vi "콜라 자판기(생산자소비자).vi"() -> ()   [LabVIEW 2018]
panel:
  out "Count Up":i32
  in  "종료":bool
  in  "반환":bool
  in  "구매":bool
  in  "동전":cluster{bool, bool, bool, bool}
  out "투입 금액":dbl
  out "링":u16(ring)
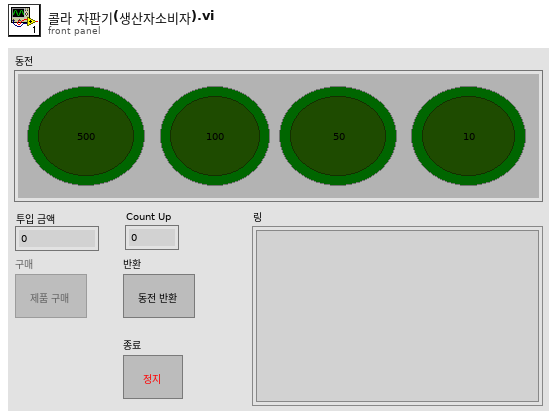
[diagram p1: front panel]
types:
  T1 = enum8{"Enabled", "Disabled", "Disabled and Grayed Out"}
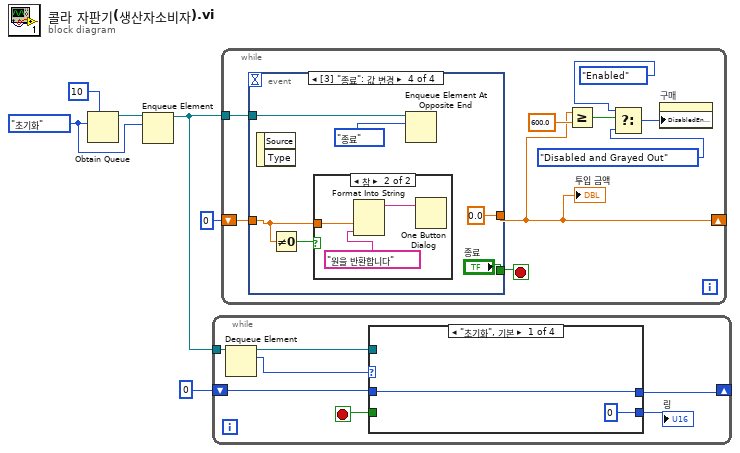
[diagram p0: block diagram]
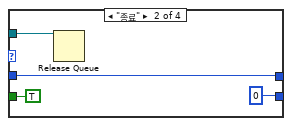
[diagram p2: hidden frame]
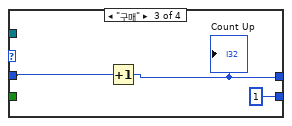
[diagram p3: hidden frame]
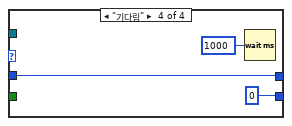
[diagram p4: hidden frame]
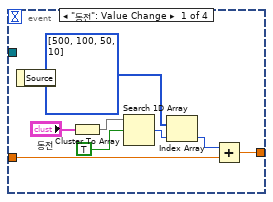
[diagram p5: hidden frame]
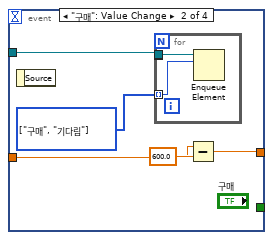
[diagram p6: hidden frame]
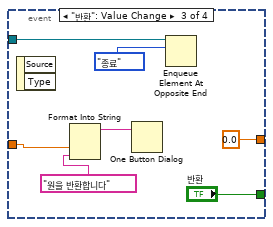
[diagram p7: hidden frame]
diagram:
  w4 = enum16{"Idle", "초기화", "종료", "구매", "반환", "기다림"}."초기화" ("열거형")
  n1 = Obtain Queue(max queue size (-1, unlimited)=10 ("최대 큐 크기(-1,제한없음)"), element data type=w4) -> (queue out=w3:refnum<queue>)  [unwired: 3 in, 2 out]
  n2 = Enqueue Element(queue=w3, element=w4) -> (queue out=w2:refnum<queue>)  [unwired: 2 in, 2 out]
  n3 = while {
    shift-right: [w8] -> _
    shift-left: 0 -> [w9]
    tunnel: w2 -> [w13]
    stop <- w7 stop-if-true
    n4 = Dequeue Element(queue=w13) -> (queue out=w11:refnum<queue>, element=w12:enum16{"Idle", "초기화", "종료", "구매", "반환", "기다림"})  [unwired: 2 in, 2 out]
    n5 = case shown="\"초기화\", 기본" w12 {
      tunnel: w11 -> [_ w18 _ _]
      tunnel: [0 0 1 0] -> w10
      tunnel: w9 -> [w14 w16 w22 w25]
      tunnel: [w14 w16 w20 w25] -> w8
      tunnel: [_ TRUE _ _] -> w7
      frame "초기화", Default {
      }
      frame "종료" {
        n6 = Release Queue(queue=w18) -> ()  [unwired: 2 in, 3 out]
      }
      frame "구매" {
        n7 = Increment(x=w22) -> (x+1=w20:i32)
        "Count Up" <- w20
      }
      frame "기다림" {
        n8 = Wait (ms)(milliseconds to wait=u32 1000 ("대기 시간 (ms)")) -> ()  [unwired: 1 out]
      }
    }
    "링" <- w10
  }
  n9 = while {
    shift-right: [w32] -> _
    shift-left: 0 -> [w34]
    tunnel: w2 -> [w27]
    stop <- w26 stop-if-true
    n10 = event shown="[3] \"종료\": 값 변경" {
      selector: _ -> [_ _ _ _]
      dyn-events: _ -> [_ _ _ _]
      timeout: _ -> [_ _ _ _]
      tunnel: [w36 w45 0.0 0.0] -> w32
      tunnel: w34 -> [w35 w46 w52 w57]
      tunnel: w27 -> [_ w44 w55 w62]
      tunnel: [_ _ "반환" "종료"] -> w26
      event "동전": Value Change {
        n11 = event-data() -> ()  [unwired: 1 in, 1 out]
        n12 = Cluster To Array(cluster="동전") -> (array=w41:bool[])
        n13 = Search 1D Array(1D array=w41, element=TRUE ("원소")) -> (index of element=w39:i32)  [unwired: 1 in]
        n14 = Index Array(array=i32[] [500, 100, 50, 10], index=w39) -> (element=w37:i32)
        n15 = Add(x=w37, y=w35) -> (x+y=w36:dbl)
      }
      event "구매": Value Change {
        w43 = enum16{"Idle", "초기화", "종료", "구매", "반환", "기다림"}[] [enum."구매", enum."기다림"] items=["Idle", "초기화", "종료", "구매", "반환", "기다림"]
        n16 = event-data() -> ()  [unwired: 1 in, 1 out]
        n17 = for {
          tunnel: [w49] -> _ mode=indexing
          tunnel: w44 -> [w49]
          tunnel: w43 -> [w48] mode=indexing
          n18 = Enqueue Element(queue=w49, element=w48) -> ()  [unwired: 2 in, 3 out]
        }
        n19 = Subtract(x=w46, y=600.0) -> (x-y=w45:dbl)
      }
      event "반환": Value Change {
        n20 = event-data() -> ()  [unwired: 1 in, 2 out]
        n21 = Format Into String(w52, "원을 반환합니다") -> (resulting string=w50:string)  [unwired: 3 in, 1 out]
        n22 = One Button Dialog(message=w50) -> ()  [unwired: 1 in, 1 out]
        n23 = Enqueue Element At Opposite End(queue=w55, element=enum16{"Idle", "초기화", "종료", "구매", "반환", "기다림"}."종료" ("열거형")) -> ()  [unwired: 2 in, 3 out]
      }
      event "종료": Value Change {
        n24 = event-data() -> ()  [unwired: 1 in, 2 out]
        n25 = Not Equal To 0?(x=w57) -> (x != 0?=w58:bool)
        n26 = case shown="참" w58 {
          tunnel: w57 -> [_ w65]
          frame False {
          }
          frame True {
            n27 = Format Into String(w65, "원을 반환합니다") -> (resulting string=w63:string)  [unwired: 3 in, 1 out]
            n28 = One Button Dialog(message=w63) -> ()  [unwired: 1 in, 1 out]
          }
        }
        n29 = Enqueue Element At Opposite End(queue=w62, element=enum16{"Idle", "초기화", "종료", "구매", "반환", "기다림"}."종료" ("열거형")) -> ()  [unwired: 2 in, 3 out]
      }
    }
    "투입 금액" <- w32
    n30 = Greater Or Equal?(x=w32, y=600.0) -> (x >= y?=w31:bool)
    n31 = Select(t=T1."Enabled" ("비활성화"), s=w31, f=T1."Disabled and Grayed Out" ("비활성화")) -> (s? t:f=w30:T1)
    n32 = property on="구매" class="Bool"("DisabledEnum"=w30) -> ()  [unwired: 2 in, 2 out]
  }
